vi "Logger Close.vi"(8 "error in (no error)":errorcluster, 10 "Ignore Remaining Elements (f)":bool, 11 "LoggerRef In":T1) -> ()   [LabVIEW 2014]
uses:
  LoggerRef.ctl
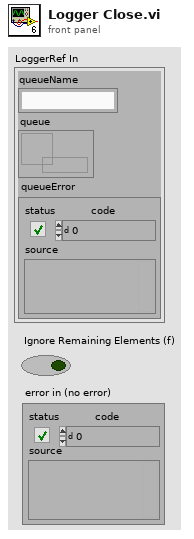
[diagram p1: front panel]
types:
  T1 = typedef "LoggerRef.ctl" = cluster{"queueName":string, "queue":refnum<queue>, "queueError":errorcluster}
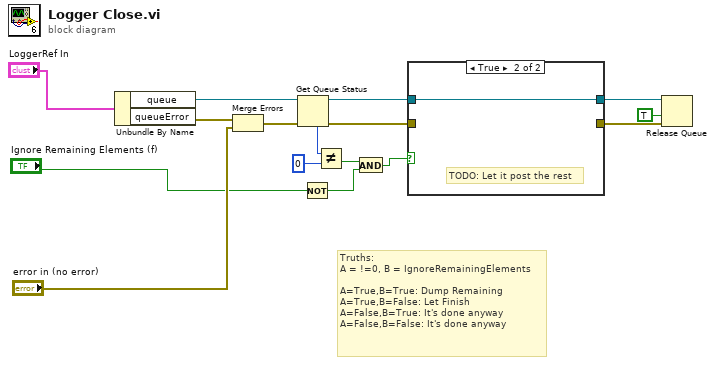
[diagram p0: block diagram]
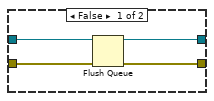
[diagram p2: hidden frame]
diagram:
  # "Truths:\nA = !=0, B = IgnoreRemainingElements\n\nA=True,B=True: Dump Remaining\nA=True,B=False: Let Finish\nA=False,B=True: It's done anyway\nA=False,B=False: It's done anyway"
  n1 = Unbundle By Name("LoggerRef In") -> ("queue"=w15:refnum<queue>, "queueError"=w14:errorcluster)
  n2 = Merge Errors(w14, "error in (no error)") -> (w12:errorcluster)
  n3 = Get Queue Status(queue=w15, error in (no error)=w12) -> (queue out=w10:refnum<queue>, error out=w9:errorcluster, # elements in queue=w11:i32)  [unwired: 1 in, 5 out]
  n4 = Not(x="Ignore Remaining Elements (f)") -> (.not. x?=w5:bool)
  n5 = Not Equal?(x=w11, y=0) -> (x != y?=w8:bool)
  n6 = And(x=w8, y=w5) -> (x .and. y?=w7:bool)
  n7 = case shown="True" w7 {
    tunnel: w10 -> [w17 w21]
    tunnel: w9 -> [w18 _]
    tunnel: [w20 w21] -> w3
    tunnel: [w19 _] -> w2
    frame False {
      n8 = Flush Queue(queue=w17, error in (no error)=w18) -> (queue out=w20:refnum<queue>, error out=w19:errorcluster)  [unwired: 1 out]
    }
    frame True {
      # "TODO: Let it post the rest"
    }
  }
  n9 = Release Queue(queue=w3, force destroy? (F)=TRUE, error in (no error)=w2) -> ()  [unwired: 3 out]
